vi "OperationCall.vi"(0 "Divide in":refnum<class "Divide.lvclass">, 5 "Sub Panel":refnum<vi>, 7 "user event out":refnum<user-event>, 9 "event source":refnum<user-event>, 11 "error in (no error)":errorcluster) -> (4 "Divide out":refnum<class "Divide.lvclass">, 15 "error out":errorcluster)   [LabVIEW 2023, in "Divide.lvclass"]
uses:
  Divide.lvclass
  Arithmetic/Arithmetic.lvclass
  SubPanelDivide.vi
  Divide.lvclass/Divide.ctl
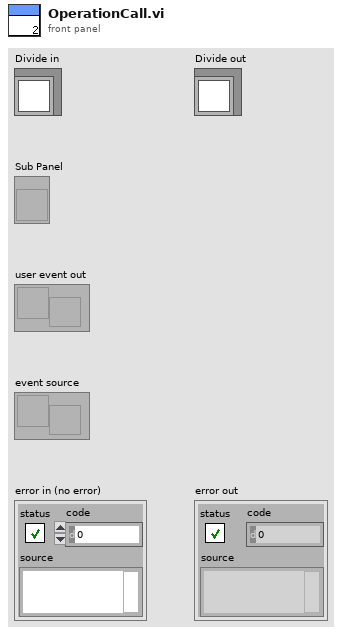
[diagram p1: front panel]
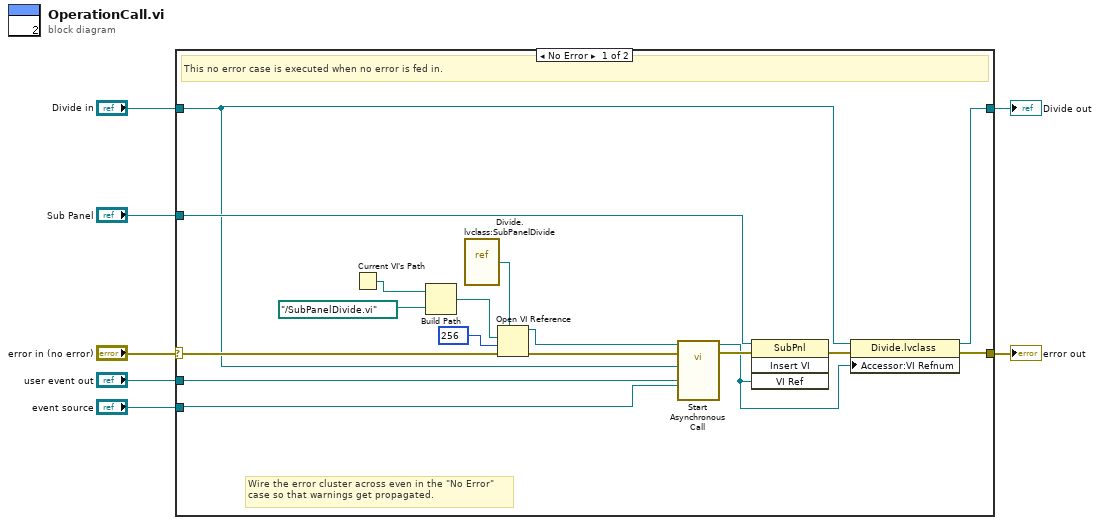
[diagram p0: block diagram]
diagram:
  n1 = case shown="No Error" "error in (no error)" {
    selector: "error in (no error)" -> [w16 w26]
    tunnel: [w11 w26] -> w6
    tunnel: [w10 w25] -> w4
    tunnel: "Divide in" -> [w8 w25]
    tunnel: "Sub Panel" -> [w13 _]
    tunnel: "user event out" -> [w15 _]
    tunnel: "event source" -> [w12 _]
    frame No Error {
      # "Wire the error cluster across even in the \"No Error\"\ncase so that warnings get propagated."
      # "This no error case is executed when no error is fed in."
      n2 = Current VI's Path() -> (path=w14:path)
      n3 = Build Path(base path=w14, name or relative path=path "../SubPanelDivide.vi") -> (appended path=w21:path)
      n4 = vi-ref "Divide.lvclass:SubPanelDivide.vi"() -> (w20:refnum<vi>)
      n5 = Open VI Reference(type specifier VI Refnum (for type only)=w20, vi path=w21, options=256, error in (no error)=w16) -> (vi reference=w18:refnum<vi>, error out=w22:errorcluster)  [unwired: 2 in]
      n6 = call-by-ref "Start Asynchronous Call"(reference=w18, error in=w22, "Divide in"=w8, "user event out"=w15, "event source"=w12) -> (reference out=w9:refnum<vi>, error out=w23:errorcluster)  [unwired: 10 in, 3 out]
      n7 = invoke on="Invoke Node" class="SubPnl" method="Insert VI"(reference=w13, error in=w23, "VI Ref"=w9) -> (error out=w17:errorcluster)  [unwired: 1 in, 3 out]
      n8 = property class="Divide.lvclass"(reference=w8, error in=w17, "Accessor:VI Refnum"=w9) -> (reference out=w10:refnum<class "Divide.lvclass">, error out=w11:errorcluster)
    }
    frame Error {
      # "This error case is executed when error is fed in and fed out through error out."
    }
  }
  "error out" <- w6
  "Divide out" <- w4
